vi "Read PLC Config.vi"(8 "error in (no error)":errorcluster, 11 "PLC in":refnum<class "MB PLC Client.lvclass">) -> (0 "error out":errorcluster, 2 "Config":T1={"Use TCP"=FALSE, "Reference Format"=4, "Swap Words"=FALSE, "Poll List"=[]} {"Reference Format" items=["4 Digits"=4, "5 Digits"=5, "6 Digits"=6]}, 3 "PLC out":refnum<class "MB PLC Client.lvclass">)   [LabVIEW 2018, in "MB PLC Client.lvlib" / "MB PLC Client.lvclass"]
uses:
  MB PLC Client.lvclass
  Types/PLC Config_Cluster.ctl
  Types/MB Ref Range_Cluster.ctl
  MB PLC Client.lvclass/MB PLC Client.ctl
  MB PLC Client.lvlib
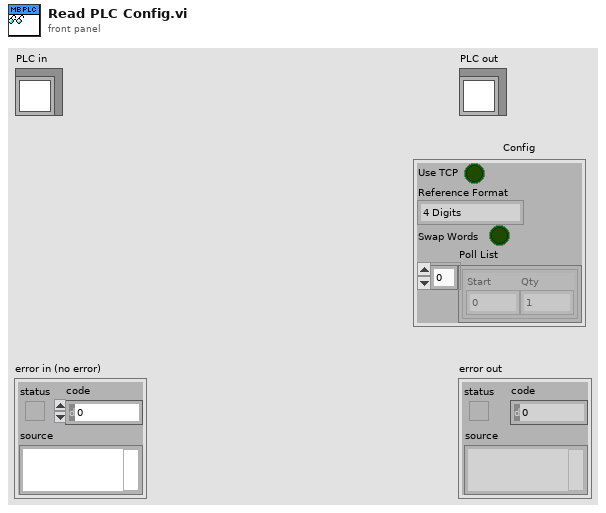
[diagram p1: front panel]
types:
  T1 = typedef "MB PLC Client.lvlib/PLC Config_Cluster.ctl" = cluster{"Use TCP":bool, "Reference Format":u16, "Swap Words":bool, "Poll List":T2[]}
  T2 = typedef "MB PLC Client.lvlib/MB Ref Range_Cluster.ctl" = cluster{"Start":u32, "Qty":u16}
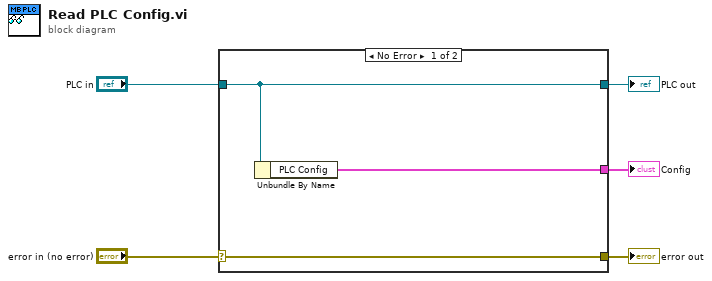
[diagram p0: block diagram]
diagram:
  n1 = case shown="No Error" "error in (no error)" {
    selector: "error in (no error)" -> [w8 w9]
    tunnel: [w8 w9] -> w4
    tunnel: [w7 w10] -> w2
    tunnel: "PLC in" -> [w7 w10]
    tunnel: [w6 _] -> w1
    frame No Error {
      n2 = Unbundle By Name(w7) -> ("PLC Config"=w6:T1)
    }
    frame Error {
    }
  }
  "error out" <- w4
  "PLC out" <- w2
  "Config" <- w1
